vi "Wrapper.vi"(10 "Accessors:CVT Session":T1, 11 "Initialize Alicat SP MSG in":refnum<class "Initialize Device SP MSG.lvclass">) -> (0 "error out":errorcluster)   [LabVIEW 2017, in "Controller.lvlib" / "Initialize Device SP MSG.lvclass"]
uses:
  Initialize Device SP MSG.lvclass
  <vilib>/MSR Consulting, LLC/General Reuse/Session APIs/_Session Fwk/Typedefs/Session Handle.ctl
  <vilib>/MSR Consulting, LLC/General Reuse/Session APIs/_Session Fwk/Session - Root.lvclass
  C:/Program Files (x86)/National Instruments/LabVIEW 2017/vi.lib/MSR Consulting, LLC/Devices/DAQ Device/Messages/Generic CVT Init/Generic Init CVT Message.lvclass
  <vilib>/MSR Consulting, LLC/Devices/DAQ Device/Messages/Generic CVT Init/Generic Init CVT Message.lvclass/Generic Init CVT Message.ctl
  <vilib>/MSR Consulting, LLC/Devices/DAQ Device/Messages/Generic CVT Init/Read DevID.vi
  <vilib>/MSR Consulting, LLC/Devices/DAQ Device/Messages/Generic CVT Init/Read SP.vi
  <vilib>/MSR Consulting, LLC/General Reuse/Session APIs/CVT/CVT.lvclass
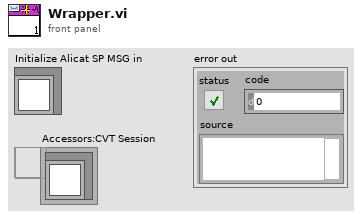
[diagram p1: front panel]
types:
  T1 = typedef "Session - Root.lvclass/Session Handle.ctl" = refnum<data-value>
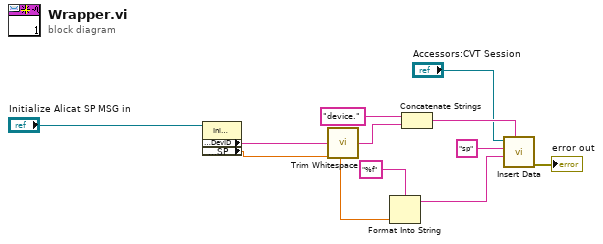
[diagram p0: block diagram]
diagram:
  n1 = property class="Initialize Alicat SP MSG"(reference="Initialize Alicat SP MSG in") -> ("Accessors:DevID"=w9:string, "Accessors:SP"=w3:dbl)  [unwired: 1 in, 2 out]
  n2 = call <vilib>:"Trim Whitespace.vi"("string"=w9) -> ("trimmed string"=w10:string)  [unwired: 1 in]
  n3 = Format Into String(format string="%f", w3) -> (resulting string=w1:string)  [unwired: 2 in, 1 out]
  n4 = Concatenate Strings("device." ("Group"), w10) -> (w7:string)
  n5 = call <vilib>:"Insert Data.vi"("Group"=w7, "Data"=w1, "tag"="sp", "CVT Session In"="Accessors:CVT Session") -> ("error out"=→"error out":errorcluster)  [unwired: 6 in, 1 out]
